vi "HFRR ADV v037 new software.vi"() -> ()   [LabVIEW 2025] (continued)
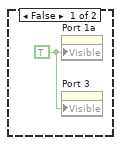
[diagram p5: hidden frame]
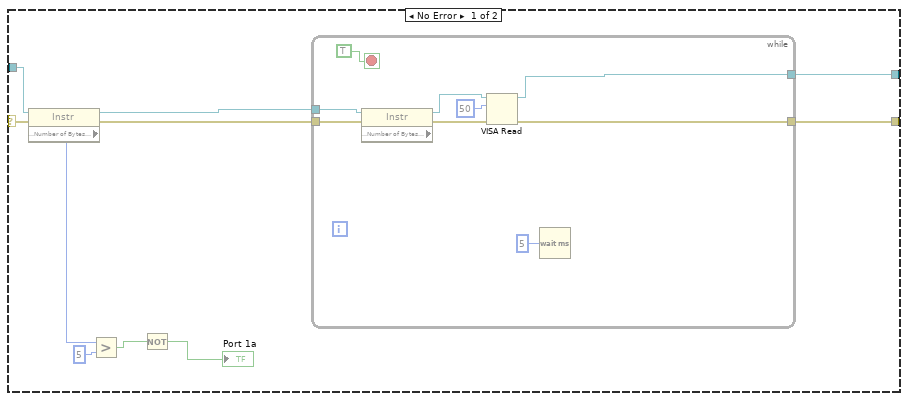
[diagram p6: hidden frame]
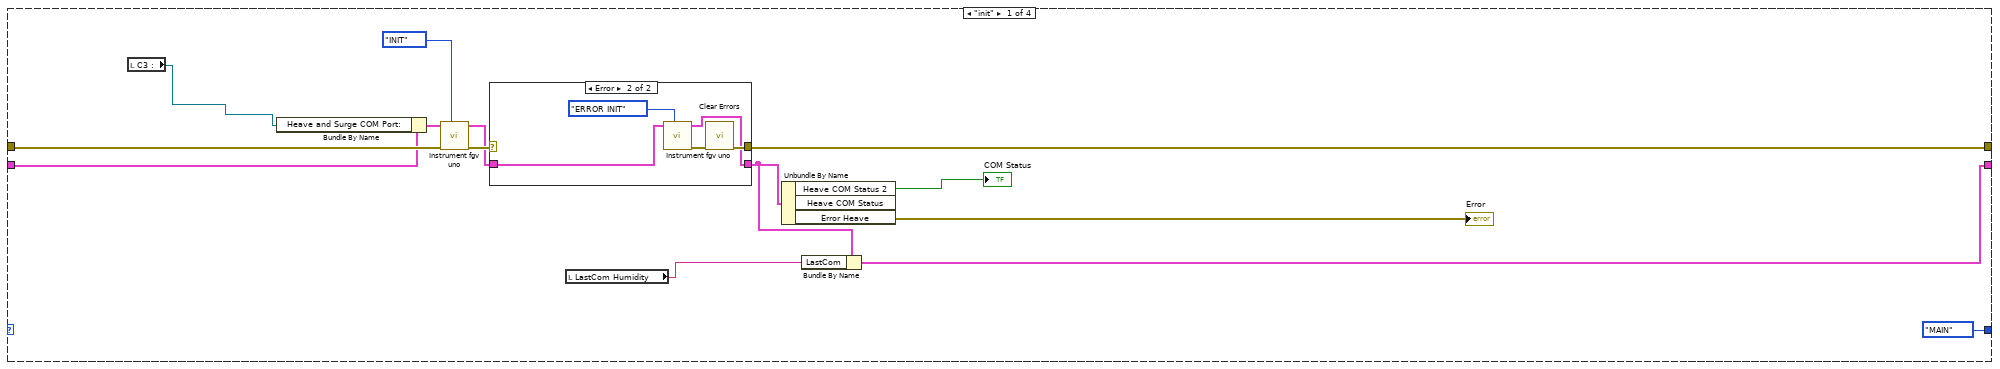
[diagram p8: hidden frame]
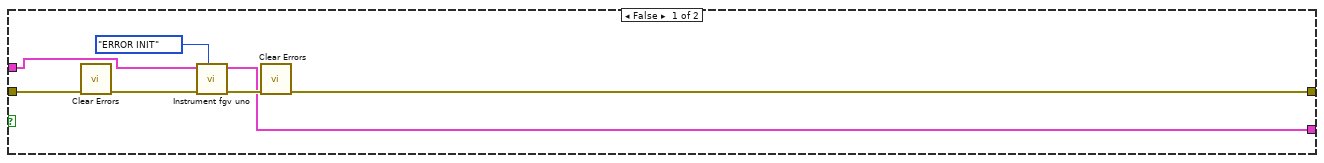
[diagram p10: hidden frame]
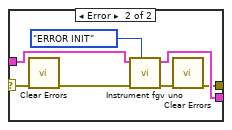
[diagram p12: hidden frame]
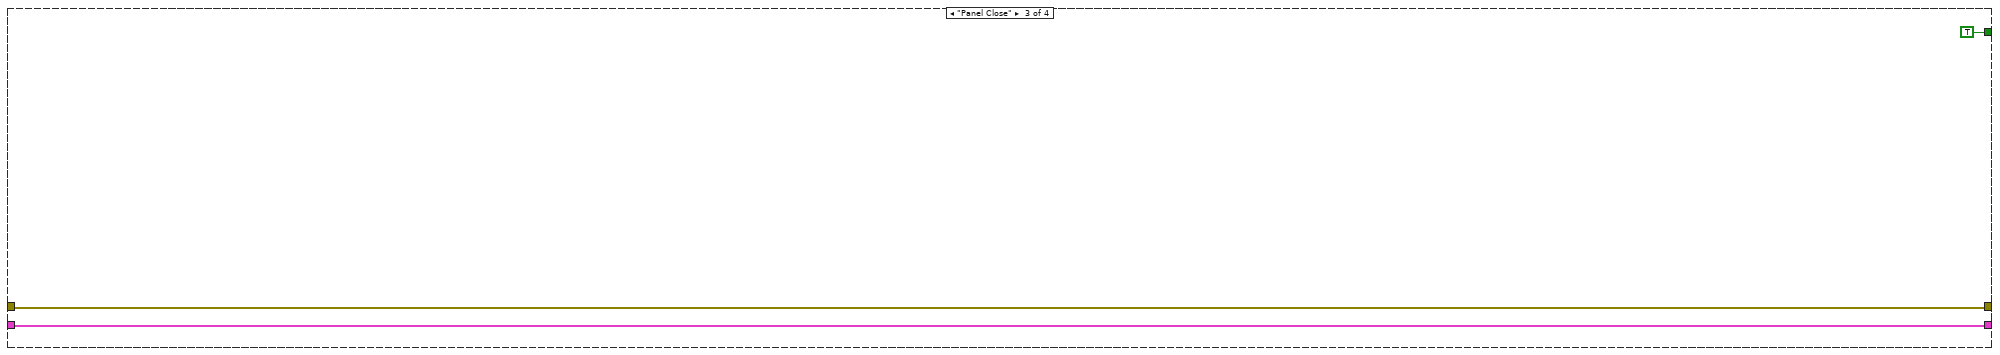
[diagram p14: hidden frame]
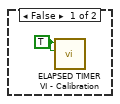
[diagram p18: hidden frame]
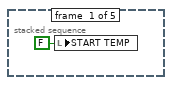
[diagram p20: hidden frame]
                n3369 = call "Instrument fgv uno.vi"("Enum"=T31."ERROR INIT", "error in (no error) 2"=w4399, "INPUT"=w4405) -> ("error"=w4403:errorcluster, "output"=w4404:T18)  [unwired: 6 in, 1 out]
                n3370 = call <vilib>:"Clear Errors.vi"("error in (no error)"=w4403) -> ("error out"=w4402:errorcluster)  [unwired: 5 in, 1 out]
              }
            }
            n3371 = Unbundle By Name(w4387) -> ("LastCom"=→"LastCom Humidity":string, "Read Heave and Surge"=→"Read HUMIDITY":string)
          }
        }
        n3372 = Unbundle By Name(w4364) -> ("Heave COM Status 2"=w4365:bool, "Error Heave"=w4353:errorcluster, "Bytes at Heave Port"=→"Bytes at Humidity Port  2":dbl)  [unwired: 1 out]
        n3373 = Unbundle By Name(w4353) -> ("status"=→"Humidity Port":bool)
        n3374 = Not(x=w4365) -> (.not. x?=w4354:bool)
        n3375 = local write "Error"(w4353) -> ()
        n3376 = local read "Quit"() -> (w4357:bool)
        n3377 = local write "COM Status"(w4354) -> ()
        n3378 = Select(t=enum16{"init", "MAIN", "Panel Close"}."Panel Close", s=w4357, f=enum16{"init", "MAIN", "Panel Close"}."MAIN") -> (s? t:f=w4356:enum16{"init", "MAIN", "Panel Close"})
      }
      frame "Panel Close" {
      }
      frame Default {
      }
    }
  }
  n3379 = while {
    stop <- w4422 stop-if-true
    n3380 = call <vilib>:"High Resolution Polling Wait.vi"("seconds to wait"=0.05) -> ()  [unwired: 10 in, 1 out]
    n3381 = disable-structure shown="Disabled" {
      disable-tunnel: [_ w4453] -> w4420
      frame Disabled {
        n3382 = local read "Read HUMIDITY"() -> (w4423:string)
        n3383 = Spreadsheet String To Array(delimiter (Tab)=",", format string="", spreadsheet string=w4423, array type (2D Dbl)=string[] []) -> (array=w4442:string[])
        n3384 = for {
          tunnel: w4442 -> [w4451] mode=indexing
          tunnel: string[] ["STATE;", "SET;", "RH;", "T;", "AMB_RH;", "AMB_T;", "PUMP;", "FAN_IN;", "FAN_OUT;", "DEHUM;", "CURRENT;", "STALL;"] -> [w4450] mode=indexing
          tunnel: [w4449] -> w4441 mode=indexing
          n3385 = Match Pattern(string=w4451, regular expression=w4450) -> (after substring=w4449:string)  [unwired: 1 in, 3 out]
        }
        n3386 = Index Array(array=w4441) -> (element #1=→"STATE :":string, element #2=→"SET :":string, element #3=w4431:string, element #4=→"T :":string, element #5=w4429:string, element #6=→"AMB_T :":string, element #7=→"PUMP :":string, element #8=→"FAN_IN :":string, element #9=→"FAN_OUT :":string, element #10=→"DEHUM :":string, element #11=→"CURRENT :":string, element #12=→"STALL :":string)  [unwired: 12 in]
        "RH :" <- w4431
        "AMB_RH :" <- w4429
        n3387 = Fract/Exp String To Number(string=w4431) -> (number=w4424:dbl)  [unwired: 3 in, 1 out]
        n3388 = Fract/Exp String To Number(string=w4429) -> (number=w4428:dbl)  [unwired: 3 in, 1 out]
        n3389 = local write "Ambient Humidity :"(w4428) -> ()
        n3390 = Equal?(x=w4424, y=0.0) -> (x = y?=w4426:bool)
        n3391 = case shown="True" w4426 {
          tunnel: [w4447 w4448] -> w4425
          tunnel: w4424 -> [w4447 _]
          frame False {
            (unwired) 0.0
            "Humidity temp" <- w4447
          }
          frame True {
            n3392 = local read "Humidity temp"() -> (w4448:dbl)
          }
        }
        "RH Numeric:" <- w4425
      }
      frame Enabled {
        n3393 = local read "Read HUMIDITY"() -> (w4474:string)
        n3394 = Spreadsheet String To Array(delimiter (Tab)=",", format string="", spreadsheet string=w4474, array type (2D Dbl)=dbl[] []) -> (array=w4470:dbl[])
        n3395 = Index Array(array=w4470) -> (element #1=→"STATE :":dbl, element #2=→"SET :":dbl, element #3=w4455:dbl, element #4=→"RH :":dbl, element #5=→"T :":dbl, element #6=→"AMB_RH :":dbl, element #7=→"AMB_T :":dbl, element #8=→"PUMP :":dbl, element #9=→"FAN_IN :":dbl, element #10=→"FAN_OUT :":dbl, element #11=→"DEHUM :":dbl, element #12=→"CURRENT :":dbl, element #13=→"STALL":dbl)  [unwired: 13 in]
        "RH Numeric:" <- w4455
        n3396 = Equal?(x=w4455, y=0.0) -> (x = y?=w4458:bool)
        n3397 = case shown="False" w4458 {
          tunnel: [w4475 w4476] -> w4454
          tunnel: w4455 -> [w4475 _]
          frame False {
            "Humidity temp 2" <- w4475
          }
          frame True {
            n3398 = local read "Humidity temp 2"() -> (w4476:dbl)
          }
        }
        n3399 = call <vilib>:"Median Filter PtByPt.vi"("rank"=2, "x"=w4454) -> ("Filtered x"=w4453:dbl)  [unwired: 2 in, 1 out]
      }
    }
    n3400 = local write "RH Numeric:"(w4420) -> ()
    n3401 = local read "Quit"() -> (w4422:bool)
  }
  n3402 = while {
    shift-right: [w4482] -> _
    shift-left: _ -> [w4483]
    shift-right: [w4480] -> _
    shift-left: T20 {"Read Uno"="", "Bytes at Heave Port"=0.0, "UNO COM Port:"="COM9", "UNO COM Port: 2"="COM7", "Residual Due"="", "UNO COM Status 2"=TRUE, "UNO COM Status"=TRUE, "Port 2"=TRUE, "Sway PPR"=6400.0, "Surge PPR"=6400.0, "Heave PPR"=6400.0, "Sway Pitch"=2.0, "Surge Pitch"=3.0, "Heave Pitch"=4.0, "Sway Pulses/mm"=320.0, "Surge Pulses/mm"=1600.0, "Heave Pulses/mm"=1600.0, "inner loop"=0.0, "Read Heave and Surge 2"="", "String 36"="", "Write S"=FALSE, "WriteCC1"=[""], "Heave COM Loop"=0, "LastCom"="", "EXIT"=FALSE, "Error Heave"={"status"=TRUE, "code"=-1073807343, "source"=""}} -> [w4479]
    shift-right: [w4477] -> _
    shift-left: enum16{"init", "MAIN", "Panel Close"}."init" -> [w4478]
    stop <- w4481 stop-if-true
    # "UNO CODE LOGIC"
    n3403 = case shown="\"MAIN\"" w4478 {
      tunnel: w4483 -> [w4497 w4516 w4572 w4574]
      tunnel: [w4492 w4521 w4572 w4574] -> w4482
      tunnel: [_ _ TRUE _] -> w4481
      tunnel: [w4488 w4519 w4570 w4573] -> w4480
      tunnel: w4479 -> [w4494 w4515 w4570 w4573]
      tunnel: [enum16{"init", "MAIN", "Panel Close"}."MAIN" w4510 _ _] -> w4477
      frame "init" {
        n3404 = local read "Com Port 1"() -> (w4484:refnum<visa-resource-name>)
        n3405 = Bundle By Name(cluster=w4494, "UNO COM Port:"=w4484) -> (w4493:T20)
        n3406 = call "Instrument fgv.vi"("Enum"=T31."INIT", "error in (no error) 2"=w4497, "INPUT"=w4493) -> ("error"=w4495:errorcluster, "output"=w4491:T18)  [unwired: 6 in, 1 out]
        n3407 = case shown="Error" w4495 {
          selector: w4495 -> [w4499 _]
          tunnel: [w4499 w4503] -> w4492
          tunnel: w4491 -> [w4498 w4501]
          tunnel: [w4498 w4500] -> w4489
          frame No Error {
          }
          frame Error {
            n3408 = call "Instrument fgv.vi"("Enum"=T31."ERROR INIT", "INPUT"=w4501) -> ("error"=w4504:errorcluster, "output"=w4500:T18)  [unwired: 7 in, 1 out]
            n3409 = call <vilib>:"Clear Errors.vi"("error in (no error)"=w4504) -> ("error out"=w4503:errorcluster)  [unwired: 5 in, 1 out]
          }
        }
        n3410 = local read "LastCom UNO"() -> (w4486:string)
        n3411 = Unbundle By Name(w4489) -> ("Heave COM Status 2"=→"Instrument Status":bool, "Error Heave"=→"Error  2":errorcluster)  [unwired: 1 out]
        n3412 = Bundle By Name(cluster=w4489, "LastCom"=w4486) -> (w4488:T18)
      }
      frame "MAIN" {
        n3413 = Unbundle By Name(w4515) -> ("UNO COM Port: 2"=w4505:refnum<visa-resource-name>)
        n3414 = local read "Com Port 1"() -> (w4506:refnum<visa-resource-name>)
        n3415 = local write "COM Port UNO :"(w4505) -> ()
        n3416 = Equal?(x=w4505, y=w4506) -> (x = y?=w4522:bool)
        n3417 = Bundle By Name(cluster=w4515, "UNO COM Port:"=w4506) -> (w4514:T20)
        n3418 = case shown="True" w4522 {
          tunnel: [w4526 w4543] -> w4521
          tunnel: w4516 -> [w4527 w4549]
          tunnel: w4514 -> [w4525 w4547]
          tunnel: [w4524 w4542] -> w4519
          frame False {
            n3419 = call <vilib>:"Clear Errors.vi"("error in (no error)"=w4527) -> ("error out"=w4523:errorcluster)  [unwired: 5 in, 1 out]
            n3420 = call "Instrument fgv.vi"("Enum"=T31."ERROR INIT", "error in (no error) 2"=w4523, "INPUT"=w4525) -> ("error"=w4529:errorcluster, "output"=w4524:T18)  [unwired: 6 in, 1 out]
            n3421 = call <vilib>:"Clear Errors.vi"("error in (no error)"=w4529) -> ("error out"=w4526:errorcluster)  [unwired: 5 in, 1 out]
          }
          frame True {
            n3422 = call "Instrument fgv.vi"("Enum"=T31."READ", "error in (no error) 2"=w4549, "INPUT"=w4547) -> ("error"=w4548:errorcluster, "output"=w4541:T18)  [unwired: 6 in, 1 out]
            n3423 = Bundle By Name(cluster=w4541, "String 36"="WRITE UNO") -> (w4540:T18)
            n3424 = case shown="True" "Write" {
              selector: "Write" -> [_ w4564]
              tunnel: w4548 -> [w4562 w4569]
              tunnel: [w4562 w4568] -> w4538
              tunnel: w4540 -> [w4561 w4566]
              tunnel: [w4561 w4565] -> w4537
              frame False {
              }
              frame True {
                n3425 = Not(x=w4564) -> (.not. x?=w4563:bool)
                n3426 = local write "Write"(w4563) -> ()
                n3427 = call "Instrument fgv.vi"("Enum"=T31."MANUAL WRITE", "error in (no error) 2"=w4569, "INPUT"=w4566) -> ("error"=w4568:errorcluster, "output"=w4565:T18)  [unwired: 6 in, 1 out]
              }
            }
            n3428 = Array Size(array="Write UNO") -> (size(s)=w4535:i32)
            n3429 = Greater Than 0?(x=w4535) -> (x > 0?=w4534:bool)
            n3430 = call "Instrument fgv.vi"("Enum"=T31."WRITE", "error in (no error) 2"=w4538, "WriteCC1"="Write UNO", "INPUT"=w4537) -> ("error"=w4545:errorcluster, "WriteCC1 2"=w4536:string[], "output"=w4544:T18)  [unwired: 5 in]
            n3431 = case shown="True" w4534 {
              tunnel: w4536 -> [_ w4551]
              frame False {
              }
              frame True {
                n3432 = local write "Write UNO"(w4551) -> ()
              }
            }
            n3433 = case shown="Error" w4545 {
              selector: w4545 -> [w4552 w4555]
              tunnel: w4544 -> [w4553 w4560]
              tunnel: [w4553 w4559] -> w4542
              tunnel: [w4552 w4557] -> w4543
              frame No Error {
              }
              frame Error {
                n3434 = call <vilib>:"Clear Errors.vi"("error in (no error)"=w4555) -> ("error out"=w4554:errorcluster)  [unwired: 5 in, 1 out]
                n3435 = call "Instrument fgv.vi"("Enum"=T31."ERROR INIT", "error in (no error) 2"=w4554, "INPUT"=w4560) -> ("error"=w4558:errorcluster, "output"=w4559:T18)  [unwired: 6 in, 1 out]
                n3436 = call <vilib>:"Clear Errors.vi"("error in (no error)"=w4558) -> ("error out"=w4557:errorcluster)  [unwired: 5 in, 1 out]
              }
            }
            n3437 = Unbundle By Name(w4542) -> ("LastCom"=→"LastCom UNO":string, "Read Heave and Surge"=→"Read UNO":string)
          }
        }
        n3438 = Unbundle By Name(w4519) -> ("Heave COM Status 2"=w4520:bool, "Heave COM Status"=w4509:bool, "Error Heave"=w4507:errorcluster, "Bytes at Heave Port"=→"Bytes at Humidity Port":dbl)
        n3439 = Not(x=w4509) -> (.not. x?=w4517:bool)
        n3440 = Not(x=w4520) -> (.not. x?=w4508:bool)
        n3441 = local write "Instrument Status"(w4517) -> ()
        n3442 = local write "Error  2"(w4507) -> ()
        n3443 = local write "Port 1a"(w4509) -> ()
        n3444 = local read "Quit"() -> (w4511:bool)
        n3445 = local write "COM Status"(w4508) -> ()
        n3446 = Select(t=enum16{"init", "MAIN", "Panel Close"}."Panel Close", s=w4511, f=enum16{"init", "MAIN", "Panel Close"}."MAIN") -> (s? t:f=w4510:enum16{"init", "MAIN", "Panel Close"})
      }
      frame "Panel Close" {
      }
      frame Default {
      }
    }
  }
